vi "GFITS_KeyPreview.vi"(6 "nd queue":bool, 7 "template path":path, 8 "error in (no error)":errorcluster, 10 "args":string, 11 "Database RefNum in":T1) -> (0 "error out":errorcluster, 2 "preview":string)   [LabVIEW 2016]
uses:
  DBSHAND/private/vis/DatabaseHand_RefNum.ctl
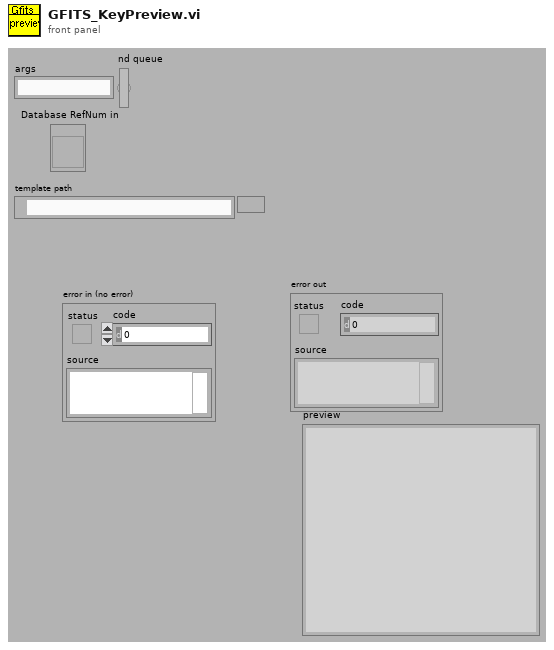
[diagram p1: front panel]
types:
  T1 = typedef "DatabaseHand_RefNum.ctl" = refnum<vi>
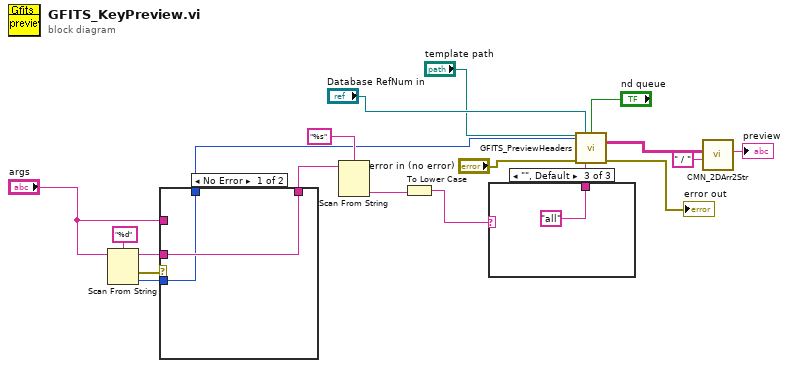
[diagram p0: block diagram]
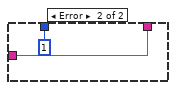
[diagram p2: hidden frame]
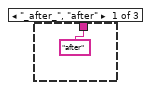
[diagram p3: hidden frame]
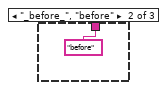
[diagram p4: hidden frame]
diagram:
  n1 = Scan From String(format string="%d", input string="args") -> (remaining string=w4:string, error out=w7:errorcluster, output 1=w6:i32)  [unwired: 2 in, 2 out]
  n2 = case shown="No Error" w7 {
    tunnel: w6 -> [w20 _]
    tunnel: [w21 w23] -> w5
    tunnel: w4 -> [w21 _]
    tunnel: [w20 1] -> w3
    tunnel: "args" -> [_ w23]
    frame No Error {
    }
    frame Error {
    }
  }
  n3 = Scan From String(format string="%s", input string=w5) -> (output 1=w18:string)  [unwired: 2 in, 4 out]
  n4 = To Lower Case(string=w18) -> (all lower case string=w17:string)
  n5 = case shown="\"\", Default" w17 {
    tunnel: ["after" "before" "all"] -> w14
    frame "_after_", "after" {
    }
    frame "_before_", "before" {
    }
    frame "", Default {
    }
  }
  n6 = call "GFITS_PreviewHeaders.vi"("file"="template path", "Database RefNum in"="Database RefNum in", "extension"=w3, "error in (no error)"="error in (no error)", "timing"=w14, "nd queue"="nd queue") -> ("headers out"=w16:string[][], "error out"=→"error out":errorcluster)  [unwired: 8 out]
  n7 = call "CMN_2DArr2Str.vi"("separator"=" / ", "array in"=w16) -> ("string out"=→"preview":string)  [unwired: 9 out]
